vi "video overlay FGV.vi"(8 "Operation":enum16{"Init", "Get", "Set"}(ring)=enum."Get", 11 "Video overlay input":dbl[](array[numeric])) -> (3 "String":string)   [LabVIEW 2021]
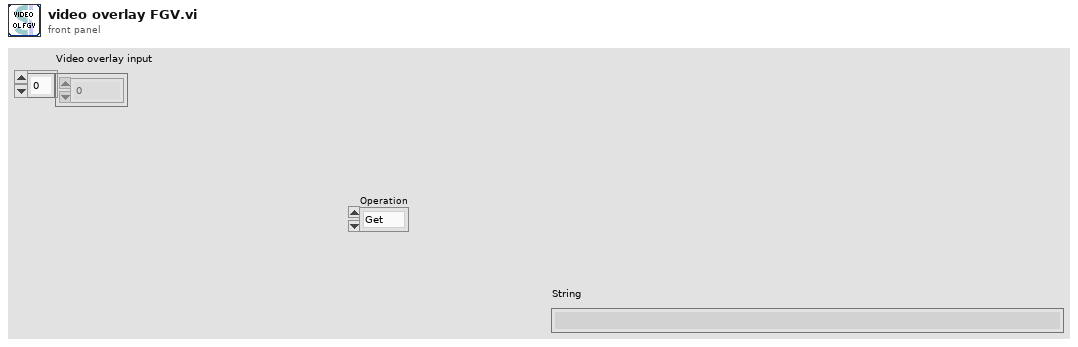
[diagram p1: front panel]
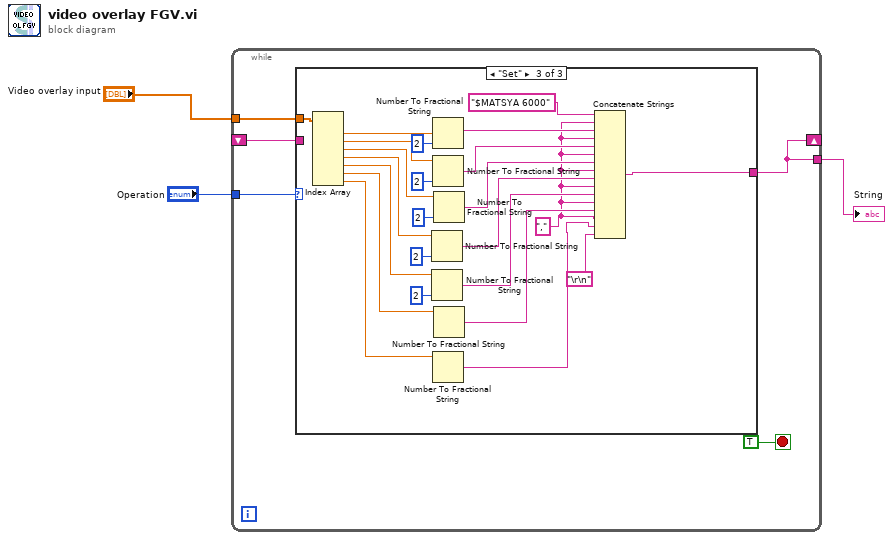
[diagram p0: block diagram]
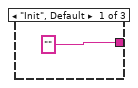
[diagram p2: hidden frame]
diagram:
  n1 = while {
    tunnel: "Operation" -> [w7]
    tunnel: "Video overlay input" -> [w6]
    tunnel: [w4] -> w2
    shift-right: [w4] -> _
    shift-left: _ -> [w5]
    stop <- TRUE stop-if-true
    n2 = case shown="\"Set\"" w7 {
      tunnel: w6 -> [_ _ w34]
      tunnel: ["" w10 w20] -> w4
      tunnel: w5 -> [_ w10 _]
      frame "Init", Default {
      }
      frame "Get" {
      }
      frame "Set" {
        w17 = ","
        n3 = Index Array(array=w34) -> (element #1=w33:dbl, element #2=w30:dbl, element #3=w28:dbl, element #4=w27:dbl, element #5=w26:dbl, element #6=w25:dbl, element #7=w19:dbl)  [unwired: 7 in]
        n4 = Number To Fractional String(number=w27, precision (6)=i16 2) -> (F-format string=w23:string)  [unwired: 2 in]
        n5 = Number To Fractional String(number=w26, precision (6)=i16 2) -> (F-format string=w22:string)  [unwired: 2 in]
        n6 = Number To Fractional String(number=w33, precision (6)=i16 2) -> (F-format string=w31:string)  [unwired: 2 in]
        n7 = Number To Fractional String(number=w30, precision (6)=i16 2) -> (F-format string=w29:string)  [unwired: 2 in]
        n8 = Number To Fractional String(number=w19) -> (F-format string=w16:string)  [unwired: 3 in]
        n9 = Number To Fractional String(number=w28, precision (6)=i16 2) -> (F-format string=w24:string)  [unwired: 2 in]
        n10 = Number To Fractional String(number=w25) -> (F-format string=w21:string)  [unwired: 3 in]
        n11 = Concatenate Strings("$MATSYA 6000" ("string"), w17, w31, w17, w29, w17, w24, w17, w23, w17, w22, w17, w21, w17, w16, "\r\n") -> (w20:string)
      }
    }
  }
  "String" <- w2
